vi "dll.midi_file_get_track_name.vi"(8 "error in (no error)":errorcluster, 10 "Track Index":i32, 11 "midi file in":refnum<class "midi file.lvclass">) -> (0 "error out":errorcluster, 2 "Track Name":string, 3 "midi file out":refnum<class "midi file.lvclass">)   [LabVIEW 2020, in "midi file.lvclass"]
uses:
  midi file.lvclass
  midi file.lvclass/midi file.ctl
  shared/midi shared.lvlib
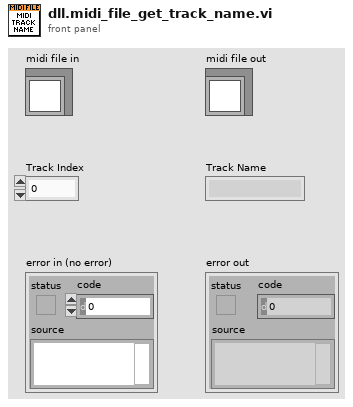
[diagram p1: front panel]
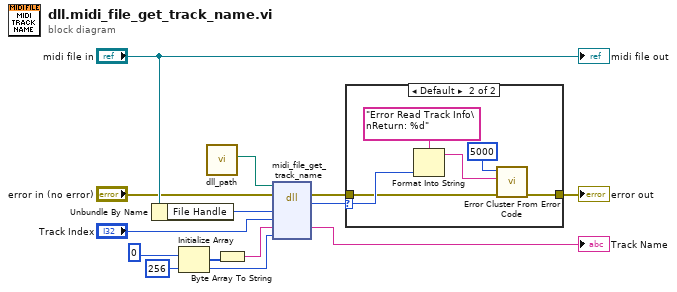
[diagram p0: block diagram]
diagram:
  w2 = 256 ("dimension size")
  n1 = Unbundle By Name("midi file in") -> ("File Handle"=w9:i32)
  n2 = Initialize Array(u8 0 ("dimension size"), w2) -> (w4:u8[])
  n3 = call "dll_path.vi"() -> ("dll"=w13:path)  [unwired: 11 in]
  n4 = Byte Array To String(unsigned byte array=w4) -> (string=w3:string)
  n5 = dll-call lib="C:/code/LabVIEW-MIDI-XPLAT/dist/TomMIDIllan_*.*" fn="midi_file_get_track_name"(path in=w13, error in="error in (no error)", "File Handle"=w9, "Track Index"="Track Index", "Buffer"=w3, "Buffer Size"=w2) -> (error out=w12:errorcluster, "Error code"=w11:i32, "Buffer"=→"Track Name":string)  [unwired: 4 in, 1 out]
  n6 = case shown="Default" w11 {
    selector: w11 -> [_ w17]
    tunnel: w12 -> [w14 w16]
    tunnel: [w14 w15] -> w7
    frame 0.. {
    }
    frame Default {
      n7 = Format Into String(format string="Error Read Track Info\nReturn: %d", w17) -> (resulting string=w18:string)  [unwired: 2 in, 1 out]
      n8 = call <vilib>:"Error Cluster From Error Code.vi"("error in (no error)"=w16, "error message (\"\")"=w18, "error code (0)"=5000) -> ("error out"=w15:errorcluster)  [unwired: 6 in]
    }
  }
  "error out" <- w7
  "midi file out" <- "midi file in"
